vi "Adder0.vi"() -> (8 "Adder0":refnum<class "Adder0.lvclass">)   [LabVIEW 2017, in "Adder0.lvclass"]
uses:
  Adder0.lvclass
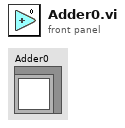
[diagram p1: front panel]
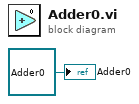
[diagram p0: block diagram]
diagram:
  "Adder0" <- refnum<class "Adder0.lvclass"> refnum ("Adder0.lvclass")
